vi "nanomsg_recv_event.vi"(4 "options":i32, 5 "level":i32, 6 "error in":errorcluster, 7 "timeout (none)":i32=-1, 8 "sockets":refnum<class "nanomsg_socket.lvclass">[](array[class]), 9 "poll event":refnum<user-event>) -> (0 "error out":errorcluster, 2 "nevents":i32, 3 "poll event out":refnum<user-event>)   [LabVIEW 2014, in "nanomsg.lvlib" / "nanomsg_socket.lvclass"]
doc: "Poll several sockets for input, and generate events when they receive data. This data can then be retrieved through an Event Structure.\n\nChecks whether each socket in <b>sockets</b> has data ready to receive, receives the data and raises an event. If no events happen within <b>timeout</b>, returns.\n\nIt is probably unsafe to use a <b>timeout</b> of 0, as if no data is received on any of the sockets, the LabVIEW process will hang indefinitely.\n\nMore details: http://sourceforge.net/p/labview-zmq/wiki/PollingAndEvents/"
uses:
  nanomsg_socket.lvclass
  poll_event_data.ctl
  poll_type.ctl
  nanomsg_poll_scalar.vi
  nanomsg.lvlib
panel:
  # "NN"
  # "labview"
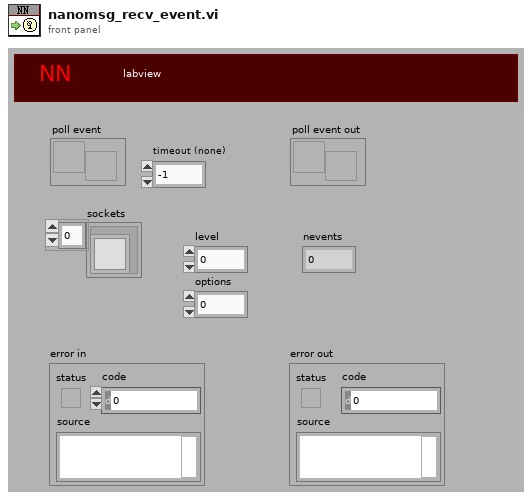
[diagram p1: front panel]
types:
  T1 = typedef "nanomsg.lvlib/poll_type.ctl" = enum16{"None", "In", "Out", "In/Out"}
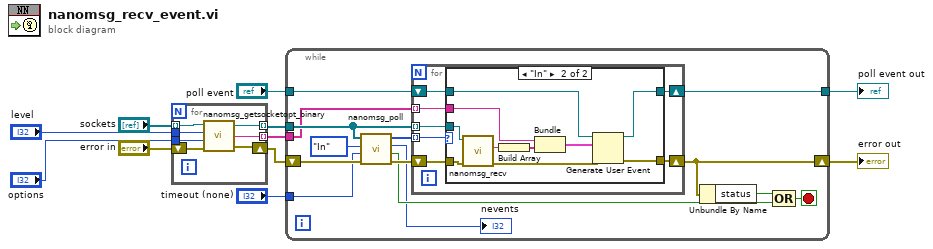
[diagram p0: block diagram]
diagram:
  n1 = for {
    tunnel: "sockets" -> [w18] mode=indexing
    shift-right: [w16] -> w5
    shift-left: "error in" -> [w17]
    tunnel: [w15] -> w3 mode=indexing
    tunnel: [w14] -> w6 mode=indexing
    tunnel: "options" -> [w13]
    tunnel: "level" -> [w12]
    n2 = call "nanomsg_getsocketopt_binary.vi"("error in"=w17, "option"=w13, "level"=w12, "socket in"=w18) -> ("error out"=w16:errorcluster, "value"=w15:string, "socket out"=w14:refnum<class "nanomsg_socket.lvclass">)
  }
  n3 = while {
    tunnel: w6 -> [w32]
    tunnel: "poll event" -> [w31]
    tunnel: [w30] -> w9
    shift-right: [w27] -> w11
    shift-left: w5 -> [w29]
    tunnel: "timeout (none)" -> [w22]
    tunnel: w3 -> [w20]
    stop <- w26 stop-if-true
    n4 = call-poly "nanomsg_poll.vi"("error in"=w29, "timeout"=w22, "poll type"=poll_type."In", "sockets"=w32) -> ("error out"=w28:errorcluster, "timed out?"=w21:bool, "nevents"=→"nevents":i32, "polled events"=w23:T1[])
    n5 = for {
      shift-right: [w38] -> w30
      shift-left: w31 -> [w39]
      shift-right: [w36] -> w27
      shift-left: w28 -> [w37]
      tunnel: w32 -> [w35] mode=indexing
      tunnel: w23 -> [w34] mode=indexing
      tunnel: w20 -> [w33] mode=indexing
      n6 = case shown="\"In\"" w34 {
        tunnel: w39 -> [w41 w51]
        tunnel: [w41 w50] -> w38
        tunnel: w37 -> [w40 w49]
        tunnel: [w40 w48] -> w36
        tunnel: w35 -> [_ w47]
        tunnel: w33 -> [_ w43]
        frame Default {
        }
        frame "In" {
          n7 = call "nanomsg_recv.vi"("error in"=w49, "socket in"=w47) -> ("error out"=w44:errorcluster, "data"=w45:string)  [unwired: 3 in, 3 out]
          n8 = Build Array(w45) -> (w42:string[])
          n9 = Bundle("value"=w43, w42) -> (w46:cluster{"value":string, string[]})  [unwired: 1 in]
          n10 = Generate User Event(user event=w51, event data cluster=w46, error in=w44) -> (user event out=w50:refnum<user-event>, error out=w48:errorcluster)  [unwired: 1 in]
        }
      }
    }
    n11 = Unbundle By Name(w27) -> ("status"=w25:bool)
    n12 = Compound Arithmetic op=OR(w25, w21) -> (w26:bool)
  }
  "error out" <- w11
  "poll event out" <- w9
